vi "LINX - PmodMIC3.vi"() -> ()   [LabVIEW 2019]
doc: "PmodMIC3\n\nThis example demonstrates how to read the voltage values from the PmodMIC3.\n\nInstructions:\n1. Select the COM Port associated with the LINX device\n2. Select the SPI Channel that the Pmod is connected to.\n3. Select the CS Channel that the Pmod is connected to.\n4. Enter the Supply Voltage used.\n5. Click the Run Arrow."
uses:
  <vilib>/MakerHub/LINX/LMH-LINX.lvlib
  <vilib>/MakerHub/LINX/Public/Sensors/Pmods/MIC3/PmodMIC3.lvlib
panel:
  out "Waveform Chart":dbl(graph)
  in  "Stop Button":bool
  in  "Serial Port":refnum<visa-resource-name>="N/A"
  out "Voltage (V)":dbl
  in  "SPI Channel (0)":u8
  in  "CS Channel":u8=10
  in  "Supply Voltage":dbl=3.3
  # "PmodMIC3\n\nThis example demonstrates how to read the voltage values from the PmodMIC3.\n\nInstructions:\n1. Select the COM Port associated with the LINX device\n2. Select the SPI Channel that the Pmod is connected to.\n3. Select the CS Channel that the Pmod is connected to.\n4. Enter the Supply Voltage used.\n5. Click the Run Arrow."
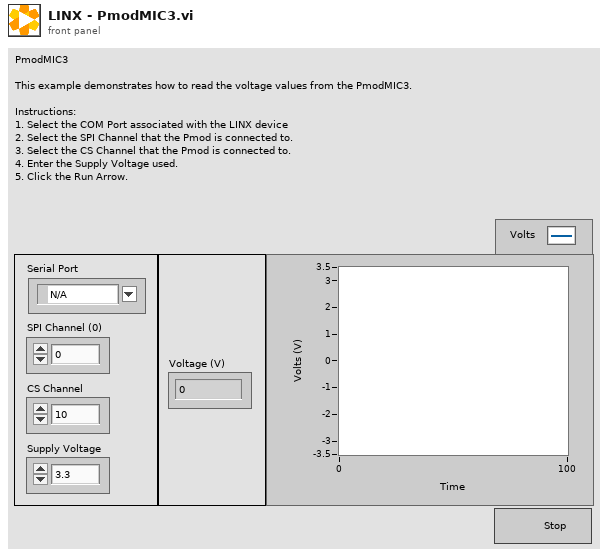
[diagram p1: front panel]
types:
  T1 = typedef "LMH-LINX.lvlib/LINX Ref.ctl" = cluster{"IO":T2, "Interface":T3, "LINX Device Config":T4}
  T2 = typedef "LMH-LINX.lvlib/Platform.ctl" = enum16{"Remote", "Local"}
  T3 = typedef "LMH-LINX.lvlib/Interface.ctl" = enum16{"Serial", "TCP"}
  T4 = typedef "LMH-LINX.lvlib/Device.lvlib/LINX Device Config.ctl" = cluster{"Interface":T3, "COM Port":refnum<visa-resource-name>, "TCP Configuration":T5, "Device Family":u8, "Device ID":u8, "Device Name":string, "TCP Ref":refnum<k5>, "Channels":T6}
  T5 = typedef "LMH-LINX.lvlib/Device.lvlib/TCP Config.ctl" = cluster{"IP Address":string, "Port":u16}
  T6 = typedef "LMH-LINX.lvlib/Channels.ctl" = cluster{"DI":u8[], "DO":u8[], "AI":u8[], "AO":u8[], "PWM":u8[], "QE":u8[], "UART":u8[], "I2C 2":u8[], "SPI":u8[], "CAN":u8[], "Servo":u8[], "AI Ref (V)":dbl, "AI Resolution (Bits)":u8, "AO Ref (V)":dbl, "AO Resolution (Bits)":u8}
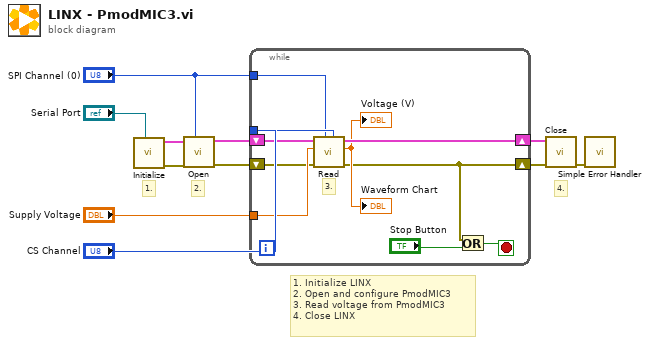
[diagram p0: block diagram]
diagram:
  # "1. Initialize LINX\n2. Open and configure PmodMIC3\n3. Read voltage from PmodMIC3\n4. Close LINX"
  # "4."
  # "2."
  # "1."
  n1 = call <vilib>:"Initialize.vi"("Serial Port"="Serial Port") -> ("Error Out"=w7:errorcluster, "LINX Resource"=w6:T1)  [unwired: 8 in, 1 out]
  n2 = call <vilib>:"Open.vi"("SPI Channel (0)"="SPI Channel (0)", "Error In"=w7, "LINX Ref"=w6) -> ("Error Out"=w8:errorcluster, "LINX Resource"=w9:T1)  [unwired: 6 in, 1 out]
  n3 = while {
    tunnel: "Supply Voltage" -> [w21]
    tunnel: "CS Channel" -> [w20]
    tunnel: "SPI Channel (0)" -> [w19]
    shift-right: [w13] -> w5
    shift-left: w8 -> [w17]
    shift-right: [w16] -> w4
    shift-left: w9 -> [w18]
    stop <- w14 stop-if-true
    # "3."
    n4 = call <vilib>:"Read.vi"("CS Channel"=w20, "SPI Channel (0)"=w19, "Error In"=w17, "Supply Voltage"=w21, "LINX Resource"=w18) -> ("Error Out"=w13:errorcluster, "Voltage (V)"=→"Voltage (V)" →"Waveform Chart":dbl, "LINX Resource"=w16:T1)  [unwired: 4 in]
    n5 = Or(x=w13, y="Stop Button") -> (x .or. y?=w14:bool)
  }
  n6 = call <vilib>:"Close.vi"("Error In"=w5, "LINX Resource"=w4) -> ("Error Out"=w3:errorcluster)  [unwired: 9 in]
  n7 = call <vilib>:"Simple Error Handler.vi"("error in (no error)"=w3) -> ()  [unwired: 4 in, 5 out]
